vi "Event Destroy.vi"(10 "Event":refnum<data-value>) -> (0 "error out":errorcluster)   [LabVIEW 2021, in "jettl Event Actor.lvlib"]
uses:
  Actor/Msg/Msg.lvclass
  jettl Event Actor.lvlib
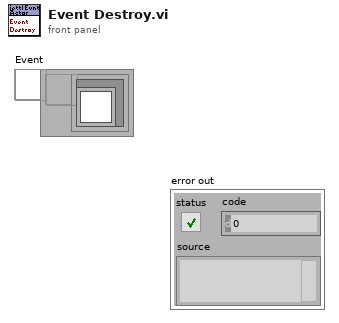
[diagram p1: front panel]
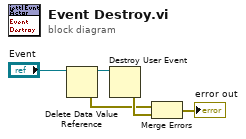
[diagram p0: block diagram]
diagram:
  n1 = Delete Data Value Reference(data value reference="Event") -> (data value=w5:refnum<user-event>, error out=w2:errorcluster)  [unwired: 1 in]
  n2 = Destroy User Event(user event=w5) -> (error out=w4:errorcluster)  [unwired: 1 in]
  n3 = Merge Errors(w2, w4) -> (→"error out":errorcluster)
